vi "Honeywell HMC6352.vi"(0 "Arduino Resource In":T1={"VISA resource"="", "Board Type"=enum."Uno", "Connection Type"=enum."USB / Serial", "Bytes Per Packet (15)"=15}, 1 "Arduino Error In":errorcluster) -> (2 "Arduino Resource Out":T1={"VISA resource"="", "Board Type"=enum."Uno", "Connection Type"=enum."USB / Serial", "Bytes Per Packet (15)"=15}, 3 "Heading (degrees)":i32, 4 "Arduino Error Out":errorcluster)   [LabVIEW 2011]
uses:
  <vilib>/LabVIEW Interface for Arduino/Type Defs/Arduino Resource.ctl
  <vilib>/LabVIEW Interface for Arduino/Type Defs/Board Type.ctl
  <vilib>/LabVIEW Interface for Arduino/LabVIEW Interface for Arduino.lvlib
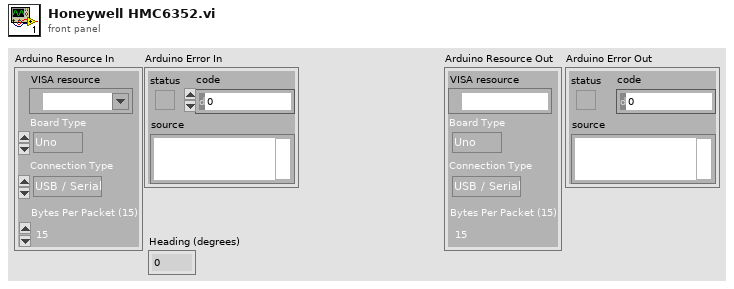
[diagram p1: front panel]
types:
  T1 = typedef "LabVIEW Interface for Arduino.lvlib/Arduino Resource.ctl" = cluster{"VISA resource":refnum<visa-resource-name>, "Board Type":T2, "Connection Type":enum8{"USB / Serial"}, "Bytes Per Packet (15)":u8}
  T2 = typedef "LabVIEW Interface for Arduino.lvlib/Board Type.ctl" = enum16{"Uno", "Dimuelanove w/Atmega 328", "Mega 2560"}
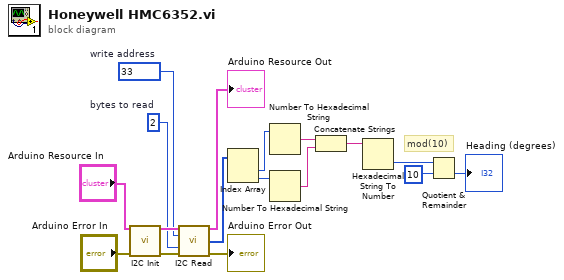
[diagram p0: block diagram]
diagram:
  w1 = u16 33  # write address
  w2 = i16 2  # bytes to read
  # "mod(10)"
  n1 = call <vilib>:"I2C Init.vi"("Arduino Resource"="Arduino Resource In", "error in"="Arduino Error In") -> ("Arduino Resource"=w8:T1, "error out"=w7:errorcluster)  [unwired: 12 in]
  n2 = call <vilib>:"I2C Read.vi"("Arduino Resource"=w8, "Address (0)"=w1, "Bytes To Read"=w2, "error in"=w7) -> ("Arduino Resource"=→"Arduino Resource Out":T1, "I2C Data"=w9:u8[], "error out"=→"Arduino Error Out":errorcluster)  [unwired: 9 in]
  n3 = Index Array(array=w9) -> (element #1=w10:u8, element #2=w11:u8)  [unwired: 2 in]
  n4 = Number To Hexadecimal String(2:w10) -> (0:w16:string)  [unwired: 1 out]
  n5 = Number To Hexadecimal String(2:w11) -> (0:w15:string)  [unwired: 1 out]
  n6 = Concatenate Strings(w16, w15) -> (w17:string)
  n7 = Hexadecimal String To Number(string=w17) -> (number=w14:u32)  [unwired: 3 out]
  n8 = Quotient & Remainder(x=w14, y=10) -> (floor(x/y)=→"Heading (degrees)":u32)  [unwired: 1 out]
